vi "oa_Modify Reset When No Tacho Pulse.vi"(9 "pulse positions [s]":dbl[](array[numeric]) format="%.2f", 10 "reset? (True)":bool=TRUE, 11 "scaled signals (EU)":waveform(dbl)[](array[waveform])) -> (2 "reset out":bool=TRUE, 3 "dup scaled signals (EU)":waveform(dbl)[](array[waveform]))   [LabVIEW 2017, in "SoundVib_Resampling.lvlib"]
uses:
  <vilib>/addons/Sound and Vibration/Order Analysis/Resample Order Tracking/SoundVib_Resampling.lvlib
  <vilib>/Waveform/WDTOps.llb/WDT Waveform Duration DBL.vi
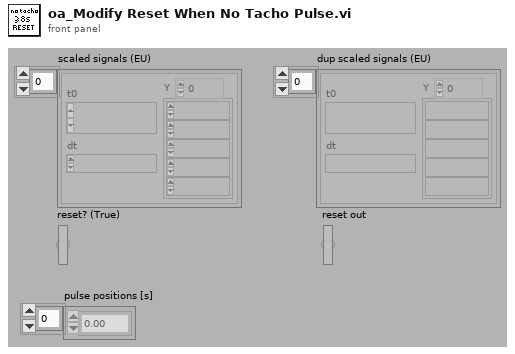
[diagram p1: front panel]
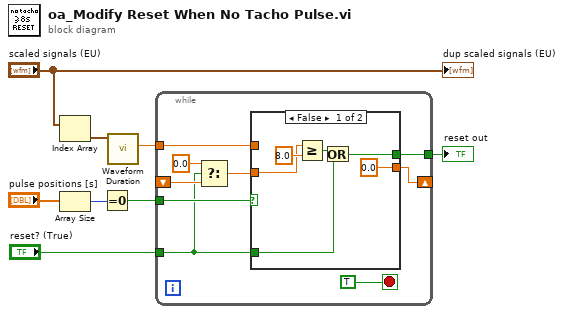
[diagram p0: block diagram]
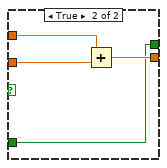
[diagram p2: hidden frame]
diagram:
  n1 = Index Array(array="scaled signals (EU)") -> (element=w7:waveform(dbl))  [unwired: 1 in]
  n2 = Array Size(array="pulse positions [s]") -> (size(s)=w5:i32)
  n3 = Equal To 0?(x=w5) -> (x = 0?=w4:bool)
  n4 = call-poly <vilib>:"Waveform Duration.vi"("waveform in"=w7) -> ("duration"=w3:dbl)  [unwired: 8 in, 2 out]
  n5 = while {
    tunnel: w4 -> [w17]
    tunnel: w3 -> [w16]
    shift-right: [w15] -> _
    shift-left: _ -> [w12]
    tunnel: "reset? (True)" -> [w11]
    tunnel: [w14] -> w1
    stop <- TRUE stop-if-true
    n6 = Select(t=0.0 ("y"), s=w11, f=w12) -> (s? t:f=w9:dbl)
    n7 = case shown="False" w17 {
      tunnel: w16 -> [_ w27]
      tunnel: w9 -> [w18 w26]
      tunnel: [0.0 w25] -> w15
      tunnel: w11 -> [w20 w24]
      tunnel: [w19 w24] -> w14
      frame False {
        n8 = Greater Or Equal?(x=w18, y=8.0) -> (x >= y?=w21:bool)
        n9 = Or(x=w21, y=w20) -> (x .or. y?=w19:bool)
      }
      frame True {
        n10 = Add(x=w27, y=w26) -> (x+y=w25:dbl)
      }
    }
  }
  "reset out" <- w1
  "dup scaled signals (EU)" <- "scaled signals (EU)"
